vi "fgv_fp-history.vi"(7 "cmd":T1, 9 "x_dr":cluster{"x":dbl, "y":dbl}, 10 "x_true":cluster{"x":dbl, "y":dbl}, 11 "x_est":cluster{"x":dbl, "y":dbl}) -> (3 "Graph sum":cluster{cluster{"x":dbl, "y":dbl}[]}[](array[cluster]))   [LabVIEW 2019]
uses:
  Ctrl/cmd_ini-RW.ctl
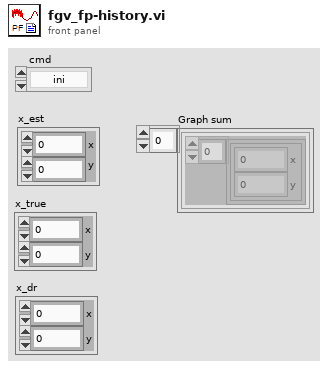
[diagram p1: front panel]
types:
  T1 = typedef "cmd_ini-RW.ctl" = enum16{"ini", "read", "write"}
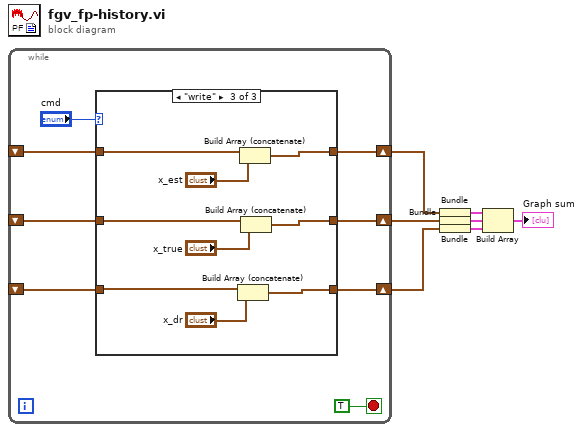
[diagram p0: block diagram]
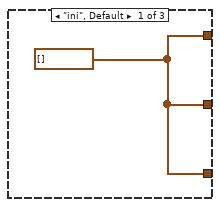
[diagram p2: hidden frame]
diagram:
  n1 = while {
    shift-right: [w13] -> w4
    shift-left: _ -> [w10]
    shift-right: [w12] -> w3
    shift-left: _ -> [w9]
    shift-right: [w11] -> w2
    shift-left: _ -> [w8]
    stop <- TRUE stop-if-true
    n2 = case shown="\"write\"" "cmd" {
      tunnel: [w16 w19 w26] -> w13
      tunnel: [w16 w18 w24] -> w12
      tunnel: [w16 w17 w21] -> w11
      tunnel: w10 -> [_ w19 w28]
      tunnel: w9 -> [_ w18 w25]
      tunnel: w8 -> [_ w17 w22]
      frame "ini", Default {
        w16 = cluster{"X":dbl, "Y":dbl}[] []
      }
      frame "read" {
      }
      frame "write" {
        n3 = Build Array (concatenate)(w22, "x_dr") -> (w21:cluster{"x":dbl, "y":dbl}[])
        n4 = Build Array (concatenate)(w28, "x_est") -> (w26:cluster{"x":dbl, "y":dbl}[])
        n5 = Build Array (concatenate)(w25, "x_true") -> (w24:cluster{"x":dbl, "y":dbl}[])
      }
    }
  }
  n6 = Bundle(w4) -> (w5:cluster{cluster{"x":dbl, "y":dbl}[]})  [unwired: 1 in]
  n7 = Bundle(w3) -> (w6:cluster{cluster{"x":dbl, "y":dbl}[]})  [unwired: 1 in]
  n8 = Bundle(w2) -> (w7:cluster{cluster{"x":dbl, "y":dbl}[]})  [unwired: 1 in]
  n9 = Build Array(w5, w6, w7) -> (→"Graph sum":cluster{cluster{"x":dbl, "y":dbl}[]}[])
